vi "Subvi sample.vi"(6 "Enable":bool, 8 "Clock":bool, 9 "Input":bool) -> (1 "Output":bool)   [LabVIEW 2017]
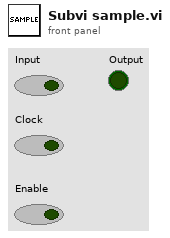
[diagram p1: front panel]
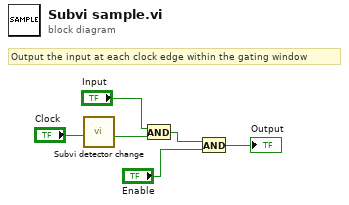
[diagram p0: block diagram]
diagram:
  # "Output the input at each clock edge within the gating window"
  n1 = call "Subvi detector change.vi"("Input"="Clock") -> ("Output"=w6:bool)  [unwired: 8 in]
  n2 = And(x="Input", y=w6) -> (x .and. y?=w3:bool)
  n3 = And(x=w3, y="Enable") -> (x .and. y?=→"Output":bool)
